vi "Launcher.vi"() -> ()   [LabVIEW 2020]
uses:
  <vilib>/Utility/miscctls.llb/LVPointTypeDef.ctl
  Controls/(Ctrl)Launcher_State Machine.ctl
  Controls/(Ctrl)Launcher_RedNoah3 Edition.ctl
  SubVIs/Control Data/Controls/(Ctrl)Control Data_Save or Load Control Data_Function.ctl
  SubVIs/Serial/Controls/(Ctrl)Serial_FGV Function.ctl
  <vilib>/Utility/sysdir.llb/System Directory Type.ctl
  SubVIs/Launcher/Controls/(Ctrl)Launcher_Edition Check form File_Function.ctl
  7ecfc601-dc53-4076-97e2-4cf976eadafe.vi
  31a6a614-1fdf-4bf0-963f-4008c2f34b95.vi
  <vilib>/security/Message Digest/API/Instances/File/SHA-256 File Checksum.vi
  <vilib>/httpClient/LabVIEWHTTPClient.lvlib
  <vilib>/zip/NI_Unzip.lvlib
  <vilib>/security/Message Digest/API/NI_Message Digest API.lvlib
panel:
  out "F/w Version":string
  out "Version":string
  out "Status":string
  # "Haptic Studio"
  # "with RedNoah3"
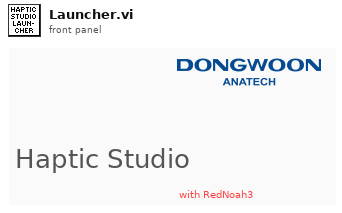
[diagram p1: front panel]
types:
  T1 = typedef "(Ctrl)Launcher_RedNoah3 Edition.ctl" = enum16{"Unknown", "Single Board", "Sensor Package"}
  T2 = typedef "(Ctrl)Launcher_State Machine.ctl" = enum16{"Check GUI Ver", "Update GUI", "Connect to BD", "Check FW Ver", "Update FW", "Check Edition", "Launch", "Server Connection Error", "BD Connection Error", "FW Update Error"}
  T3 = typedef "LVPointTypeDef.ctl" = cluster{"Horizontal":i16, "Vertical":i16}
  T4 = typedef "(Ctrl)Control Data_Save or Load Control Data_Function.ctl" = enum16{"Save", "Load"}
  T5 = cluster{"Major":i32, "Minor":i32, "Patch":i32, "Build":i32}
  T6 = typedef "(Ctrl)Serial_FGV Function.ctl" = enum16{"Initialize", "Read", "Read All", "Write", "Flush Buffer", "Get Ref.", "Close"}
  T7 = typedef "(Ctrl)Launcher_Edition Check form File_Function.ctl" = enum16{"Read", "Write"}
  T8 = enum32{"Invalid", "Standard", "Closed", "Hidden", "Minimized", "Maximized"}
  T9 = typedef "LabVIEWHTTPClient.lvlib/ClientHandle.ctl" = refnum<k1>
  T10 = typedef "Haptic IC.lvclass/(Ctrl)IC Type.ctl" = enum8{"DW7800", "DW7802", "DW7912", "DW7914"}
  T11 = cluster{"BD SN":string, "BD FW Version":u32, "BD HW Version":enum8{"BBB 1.0", "BBB 1.1", "WBB 1.0", "reserved", "RedNoah3"}}
  T12 = typedef "System Directory Type.ctl" = i32
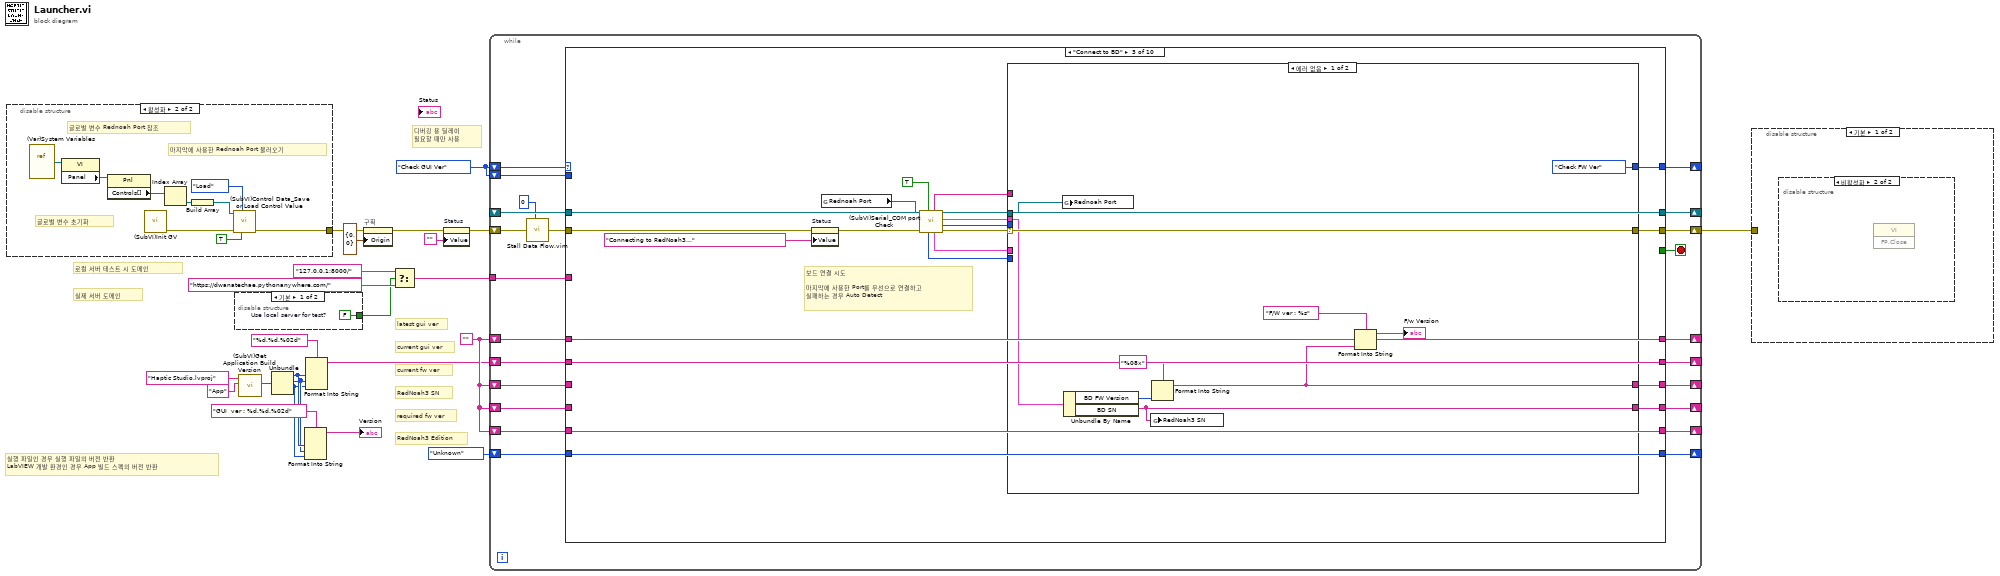
[diagram p0: block diagram]
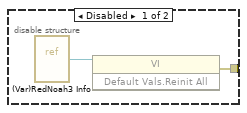
[diagram p2: hidden frame]
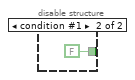
[diagram p3: hidden frame]
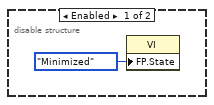
[diagram p4: hidden frame]
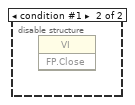
[diagram p5: hidden frame]
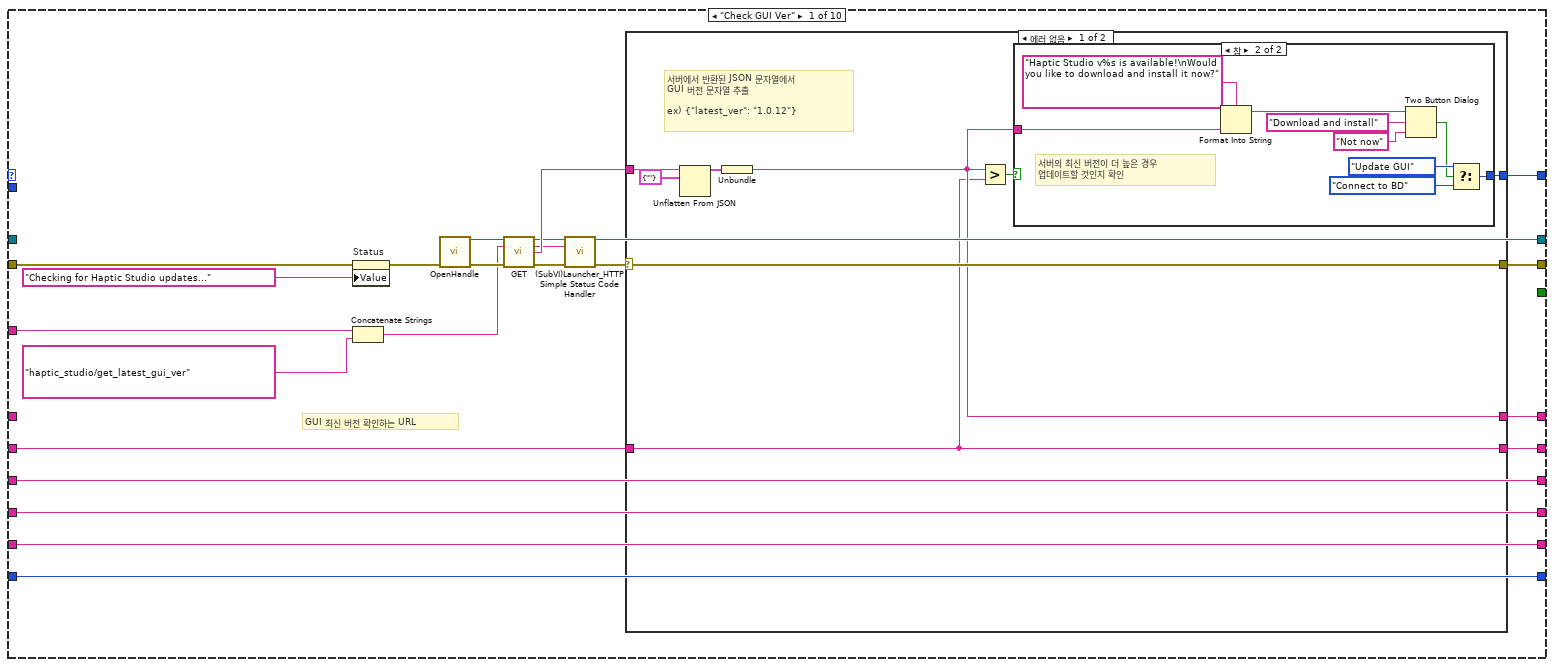
[diagram p6: hidden frame]
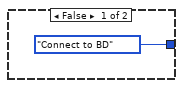
[diagram p7: hidden frame]
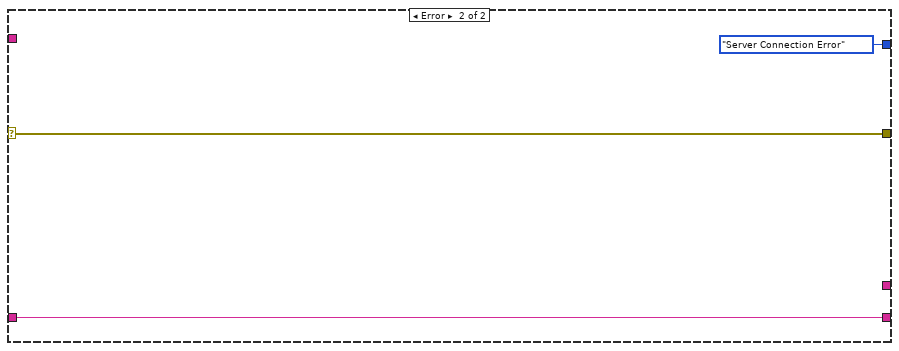
[diagram p8: hidden frame]
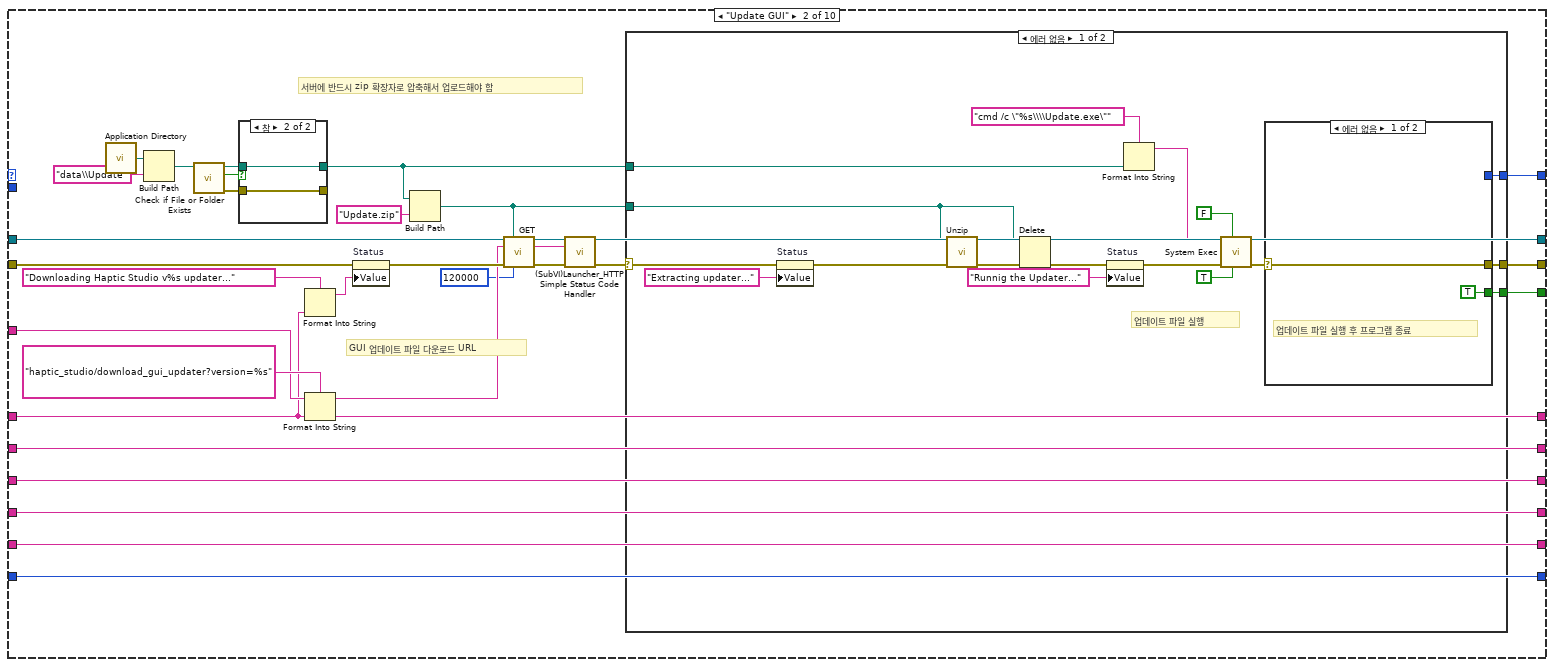
[diagram p9: hidden frame]
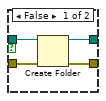
[diagram p10: hidden frame]
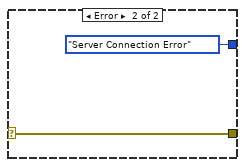
[diagram p11: hidden frame]
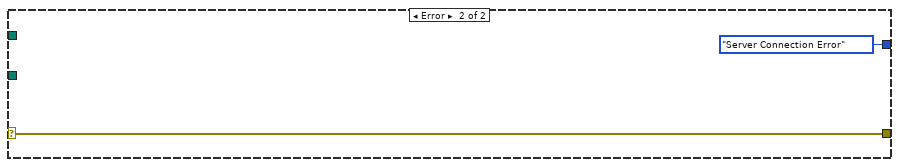
[diagram p12: hidden frame]
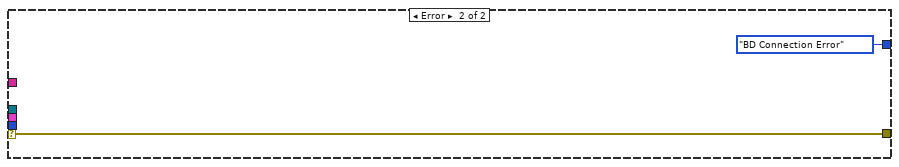
[diagram p13: hidden frame]
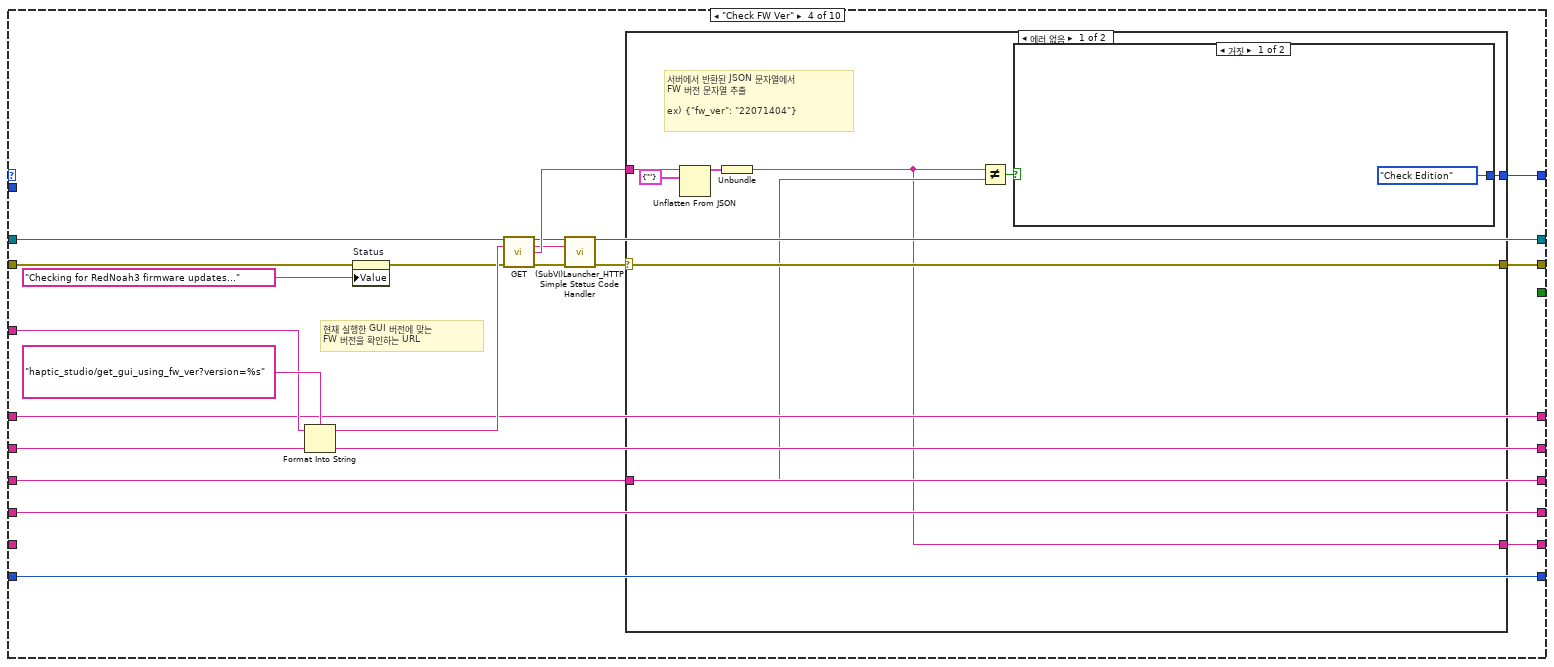
[diagram p14: hidden frame]
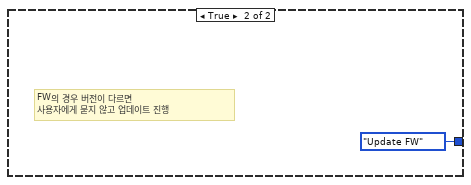
[diagram p15: hidden frame]
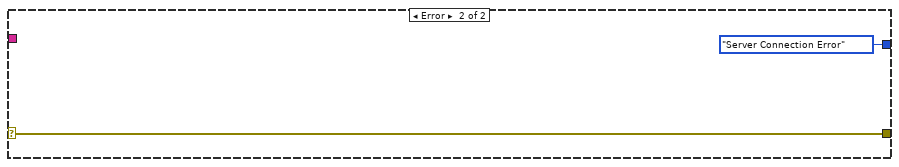
[diagram p16: hidden frame]
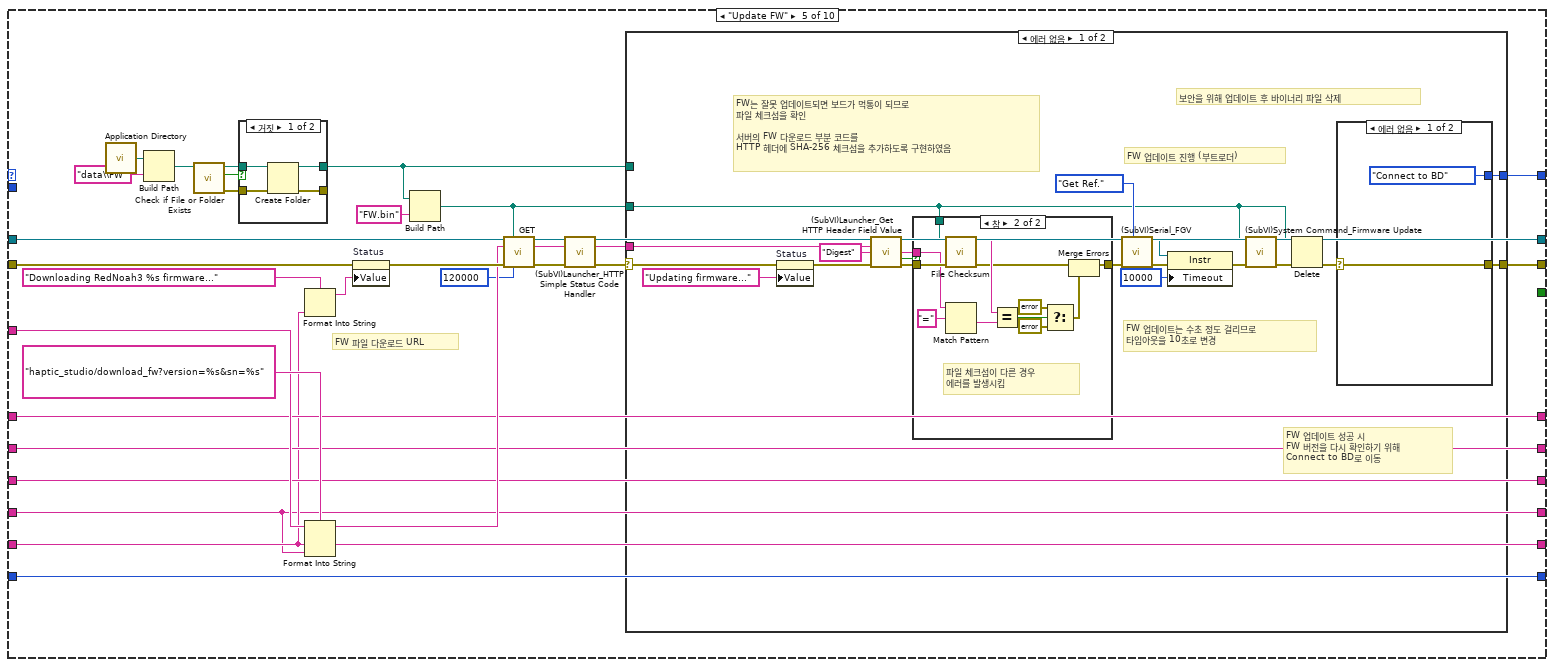
[diagram p17: hidden frame]
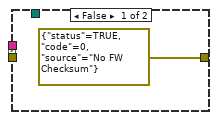
[diagram p19: hidden frame]
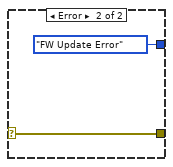
[diagram p20: hidden frame]
diagram:
  w16 = ""
  w15 = (Ctrl)Launcher_State_Machine."Check GUI Ver"
  # "실행 파일인 경우 실행 파일의 버전 반환\nLabVIEW 개발 환경인 경우 App 빌드 스펙의 버전 반환"
  # "디버깅 용 딜레이\n필요할 때만 사용"
  # "로컬 서버 테스트 시 도메인"
  # "실제 서버 도메인"
  # "RedNoah3 Edition"
  # "RedNoah3 SN"
  # "required fw ver"
  # "current fw ver"
  # "current gui ver"
  # "latest gui ver"
  n1 = disable-structure shown="활성화" {
    disable-tunnel: [w24 w33] -> w14
    frame Disabled {
      n2 = vi-ref "(Var)RedNoah3 Info.vi"() -> (w25:refnum<vi>)
      n3 = invoke class="VI" method="Default Vals.Reinit All"(reference=w25) -> (error out=w24:errorcluster)  [unwired: 2 in, 2 out]
    }
    frame Enabled {
      # "글로벌 변수 Rednoah Port 참조"
      # "마지막에 사용한 Rednoah Port 불러오기"
      # "글로벌 변수 초기화"
      n4 = vi-ref "(Var)System Variables.vi"() -> (w32:refnum<vi>)
      n5 = property class="VI"(reference=w32) -> ("Panel"=w31:refnum<vi>)  [unwired: 1 in, 2 out]
      n6 = property class="Pnl"(reference=w31) -> ("Controls[]"=w30:refnum<vi>[])  [unwired: 1 in, 2 out]
      n7 = call "(SubVI)Init GV.vi"() -> ("error out"=w34:errorcluster)  [unwired: 11 in]
      n8 = Index Array(array=w30) -> (element=w29:refnum<vi>)  [unwired: 1 in]
      n9 = Build Array(w29) -> (w28:refnum<vi>[])
      n10 = call "(SubVI)Control Data_Save or Load Control Value.vi"("Common? (f)"=TRUE, "Function"=(Ctrl)Control_Data_Save_or_Load_Control_Data_Function."Load", "error in (no error)"=w34, "Control Ref"=w28) -> ("error out"=w33:errorcluster)  [unwired: 7 in]
    }
  }
  n11 = disable-structure shown="기본" {
    disable-tunnel: [w35 FALSE ("s")] -> w19
    frame condition #0 (active) {
      w35 = FALSE  # Use local server for test?
    }
    frame condition #1 {
    }
  }
  n12 = call "(SubVI)Get Application Build Version.vi"("Build Specification Name"="App", "Project Filename"="Haptic Studio.lvproj") -> ("Version Numbers"=w10:T5)  [unwired: 7 in, 2 out]
  n13 = Unbundle(w10) -> ("Major"=w4:i32, "Minor"=w2:i32, "Patch"=w1:i32)  [unwired: 1 out]
  n14 = Format Into String(format string="GUI  ver : %d.%d.%02d" ("포맷 문자열"), w4, w2, w1) -> (resulting string=→"Version":string)  [unwired: 2 in, 1 out]
  n15 = Format Into String(format string="%d.%d.%02d" ("포맷 문자열"), w4, w2, w1) -> (resulting string=w6:string)  [unwired: 2 in, 1 out]
  n16 = property on="구획" class="Pane"(error in=w14, "Origin"=T3 {"Horizontal"=0, "Vertical"=0} ("원점")) -> (error out=w13:errorcluster)  [unwired: 1 in, 1 out]
  n17 = Select(t="127.0.0.1:8000/", s=w19, f="https://dwanatechae.pythonanywhere.com/") -> (s? t:f=w18:string)
  n18 = property on="Status" class="Str"(error in=w13, "Value"="" ("Status")) -> (error out=w11:errorcluster)  [unwired: 1 in, 1 out]
  n19 = while {
    shift-right: [w40] -> w22
    shift-left: w11 -> [w59]
    shift-right: [w57] -> _
    shift-left: _ -> [w56]
    shift-right: [w55] -> _
    shift-left: w16 -> [w54]
    shift-right: [w53] -> _
    shift-left: w15 -> [w58]
    tunnel: w18 -> [w51]
    shift-right: [w50] -> _
    shift-left: w6 -> [w49]
    shift-right: [w48] -> _
    shift-left: w16 -> [w37]
    shift-right: [w47] -> _
    shift-left: w16 -> [w46]
    shift-right: [w45] -> _
    shift-left: w16 -> [w44]
    shift-right: [w43] -> _
    shift-left: (Ctrl)Launcher_RedNoah3_Edition."Unknown" -> [w42]
    shift-left: w15 -> [w41]
    stop <- w52 stop-if-true
    n20 = call "Stall Data Flow.vim"("value in"=w59, "milliseconds to wait"=u32 0) -> ("value out"=w39:errorcluster)  [unwired: 1 out]
    n21 = case shown="\"Connect to BD\"" w58 {
      selector: w58 -> [_ _ _ _ _ _ _ w383 w401 w420]
      tunnel: w39 -> [w80 w135 w185 w218 w262 w329 w346 w387 w415 w434]
      tunnel: [w75 w132 w182 w214 w259 w324 w353 _ _ _] -> w40
      tunnel: [w62 w105 w180 w199 w234 w309 w359 w391 w419 w438] -> w57
      tunnel: w56 -> [_ w130 w180 w204 w257 _ w359 w391 w419 w438]
      tunnel: [w74 w108 w168 w207 w241 w319 w358 w390 w418 w437] -> w55
      tunnel: w54 -> [_ w108 w168 w207 w241 w319 w358 w390 w418 w437]
      tunnel: [w77 w134 w184 w216 w261 w326 _ w380 w405 w424] -> w53
      tunnel: [_ w115 _ _ _ _ TRUE _ _ _] -> w52
      tunnel: w51 -> [w73 w114 _ w212 w242 w322 _ _ _ _]
      tunnel: [w70 w113 w169 w208 w240 w317 w357 w389 w417 w436] -> w50
      tunnel: w49 -> [w60 w113 w169 w208 w240 w317 w357 w389 w417 w436]
      tunnel: [w69 w112 w171 w205 w239 w316 w352 w385 w413 w432] -> w48
      tunnel: w37 -> [w69 w112 _ w205 w239 w316 w352 w385 w413 w432]
      tunnel: [w67 w110 w167 w210 w237 w318 w356 w388 w416 w435] -> w47
      tunnel: w46 -> [w67 w110 w167 _ w237 w318 w356 w388 w416 w435]
      tunnel: [w68 w111 w170 w209 w231 w307 w351 w381 w412 w431] -> w45
      tunnel: w44 -> [w68 w111 _ w209 w231 w307 w351 w381 w412 w431]
      tunnel: [w66 w109 w166 w206 w238 w320 w350 w378 w411 w430] -> w43
      tunnel: w42 -> [w66 w109 w166 w206 w238 _ w350 w379 w411 w430]
      tunnel: w41 -> [_ _ _ _ _ _ _ w382 w402 w421]
      frame "Check GUI Ver" {
        # "GUI 최신 버전 확인하는 URL"
        n22 = property on="Status" class="Str"(error in=w80, "Value"="Checking for Haptic Studio updates..." ("Status")) -> (error out=w79:errorcluster)  [unwired: 1 in, 1 out]
        n23 = Concatenate Strings(w73, "haptic_studio/get_latest_gui_ver" ("url")) -> (w71:string)
        n24 = call <vilib>:"OpenHandle.vi"("error in (no error)"=w79) -> ("client handle out"=w82:T9, "error out"=w81:errorcluster)  [unwired: 13 in]
        n25 = call <vilib>:"GET.vi"("client handle"=w82, "url"=w71, "error in (no error)"=w81) -> ("client handle out"=w63:T9, "headers"=w61:string, "body"=w65:string, "error out"=w76:errorcluster)  [unwired: 9 in]
        n26 = call "(SubVI)Launcher_HTTP Simple Status Code Handler.vi"("client handle in"=w63, "HTTP Header"=w61, "error in (no error)"=w76) -> ("client handle out"=w62:T9, "error out"=w64:errorcluster)  [unwired: 7 in, 4 out]
        n27 = case shown="에러 없음" w64 {
          selector: w64 -> [w85 w103]
          tunnel: w65 -> [w88 _]
          tunnel: [w86 (Ctrl)Launcher_State_Machine."Server Connection Error" ("f")] -> w77
          tunnel: [w85 w103] -> w75
          tunnel: [w84 _] -> w74
          tunnel: [w83 w101] -> w70
          tunnel: w60 -> [w83 w101]
          frame No Error {
            # "서버에서 반환된 JSON 문자열에서\nGUI 버전 문자열 추출\n\nex) {\"latest_ver\": \"1.0.12\"}"
            n28 = Unflatten From JSON(JSON string=w88, type and defaults=cluster{"latest_ver":string} {"latest_ver"=""}) -> (value=w89:cluster{"latest_ver":string})  [unwired: 5 in, 1 out]
            n29 = Unbundle(w89) -> ("latest_ver"=w84:string)
            n30 = Greater?(x=w84, y=w83) -> (0:w87:bool)
            n31 = case shown="참" w87 {
              tunnel: [(Ctrl)Launcher_State_Machine."Connect to BD" ("f") w98] -> w86
              tunnel: w84 -> [_ w92]
              frame False {
              }
              frame True {
                # "서버의 최신 버전이 더 높은 경우\n업데이트할 것인지 확인"
                n32 = Format Into String(format string="Haptic Studio v%s is available!\nWould you like to download and install it now?" ("메시지"), w92) -> (resulting string=w95:string)  [unwired: 2 in, 1 out]
                n33 = Two Button Dialog(message=w95, 1:"Not now" ("거짓 버튼 이름(\"취소\")"), 2:"Download and install" ("참 버튼 이름(\"확인\")")) -> (T button?=w97:bool)
                n34 = Select(t=(Ctrl)Launcher_State_Machine."Update GUI", s=w97, f=(Ctrl)Launcher_State_Machine."Connect to BD") -> (s? t:f=w98:T2)
              }
            }
          }
          frame Error {
          }
        }
      }
      frame "Update GUI" {
        # "서버에 반드시 zip 확장자로 압축해서 업로드해야 함"
        # "GUI 업데이트 파일 다운로드 URL"
        n35 = call <vilib>:"Application Directory.vi"() -> ("Application Directory"=w125:path)
        n36 = Build Path(base path=w125, name or relative path="data\\Update" ("이름 또는 상대 경로")) -> (appended path=w123:path)
        n37 = call <vilib>:"Check if File or Folder Exists.vi"("path"=w123) -> ("error out"=w121:errorcluster, "file or folder exists?"=w122:bool, "dup path"=w120:path)  [unwired: 8 in]
        n38 = case shown="참" w122 {
          tunnel: w121 -> [w139 w141]
          tunnel: [w138 w141] -> _
          tunnel: w120 -> [w137 w140]
          tunnel: [w136 w140] -> w116
          frame False {
            n39 = Create Folder(path (use dialog)=w137, error in=w139) -> (created path=w136:path, error out=w138:errorcluster)  [unwired: 1 in, 1 out]
          }
          frame True {
          }
        }
        n40 = Format Into String(format string="Downloading Haptic Studio v%s updater..." ("Status"), w108) -> (resulting string=w128:string)  [unwired: 2 in, 1 out]
        n41 = Format Into String(format string="haptic_studio/download_gui_updater?version=%s" ("url"), initial string=w114, w108) -> (resulting string=w126:string)  [unwired: 1 in, 1 out]
        n42 = property on="Status" class="Str"(error in=w135, "Value"=w128) -> (error out=w131:errorcluster)  [unwired: 1 in, 1 out]
        n43 = Build Path(base path=w116, name or relative path="Update.zip" ("이름 또는 상대 경로")) -> (appended path=w117:path)
        n44 = call <vilib>:"GET.vi"("client handle"=w130, "output file"=w117, "url"=w126, "error in (no error)"=w131, "timeout (10000)"=120000) -> ("client handle out"=w106:T9, "headers"=w104:string, "error out"=w133:errorcluster)  [unwired: 7 in, 1 out]
        n45 = call "(SubVI)Launcher_HTTP Simple Status Code Handler.vi"("client handle in"=w106, "HTTP Header"=w104, "error in (no error)"=w133) -> ("client handle out"=w105:T9, "error out"=w107:errorcluster)  [unwired: 7 in, 4 out]
        n46 = case shown="에러 없음" w107 {
          selector: w107 -> [w150 w164]
          tunnel: [w142 (Ctrl)Launcher_State_Machine."Server Connection Error" ("f")] -> w134
          tunnel: [w143 w164] -> w132
          tunnel: w117 -> [w157 _]
          tunnel: w116 -> [w156 _]
          tunnel: [w152 _] -> w115
          frame No Error {
            # "업데이트 파일 실행"
            n47 = property on="Status" class="Str"(error in=w150, "Value"="Extracting updater..." ("Status")) -> (error out=w149:errorcluster)  [unwired: 1 in, 1 out]
            n48 = call <vilib>:"Unzip.vi"("error in (no error)"=w149, "Zip file"=w157) -> ("error out"=w158:errorcluster)  [unwired: 7 in, 2 out]
            n49 = Delete(path (use dialog)=w157, error in=w158) -> (error out=w146:errorcluster)  [unwired: 3 in, 2 out]
            n50 = property on="Status" class="Str"(error in=w146, "Value"="Runnig the Updater..." ("Status")) -> (error out=w145:errorcluster)  [unwired: 1 in, 1 out]
            n51 = Format Into String(format string="cmd /c \"%s\\\\Update.exe\"" ("포맷 문자열"), w156) -> (resulting string=w154:string)  [unwired: 2 in, 1 out]
            n52 = call <vilib>:"System Exec.vi"("run minimized? (F)"=TRUE, "wait until completion? (T)"=FALSE, "error in (no error)"=w145, "command line"=w154) -> ("error out"=w144:errorcluster)  [unwired: 4 in, 3 out]
            n53 = case shown="에러 없음" w144 {
              selector: w144 -> [w160 w162]
              tunnel: [TRUE _] -> w152
              tunnel: [w160 w162] -> w143
              tunnel: [_ (Ctrl)Launcher_State_Machine."Server Connection Error" ("f")] -> w142
              frame No Error {
                # "업데이트 파일 실행 후 프로그램 종료"
              }
              frame Error {
              }
            }
          }
          frame Error {
          }
        }
      }
      frame "Connect to BD" {
        # "보드 연결 시도\n\n마지막에 사용한 Port를 우선으로 연결하고\n실패하는 경우 Auto Detect"
        n54 = property on="Status" class="Str"(error in=w185, "Value"="Connecting to RedNoah3..." ("Status")) -> (error out=w181:errorcluster)  [unwired: 1 in, 1 out]
        n55 = global read "(Var)System Variables.vi" "Rednoah Port"() -> (w165:refnum<visa-resource-name>)
        n56 = call "(SubVI)Serial_COM port Check.vi"("Auto Detect?"=TRUE, "error in (no error)"=w181, "VISA resource name"=w165) -> ("error out"=w183:errorcluster, "IC Type"=w173:T10, "BD Version"=w175:T11, "VISA resource name out"=w174:refnum<visa-resource-name>, "I2C Slave ID"=w177:cluster{string, u8}[], "BD Info Str"=w178:string, "Default I2C Slave ID"=w176:u8)  [unwired: 2 in]
        n57 = case shown="에러 없음" w183 {
          selector: w183 -> [w194 w197]
          tunnel: [(Ctrl)Launcher_State_Machine."Check FW Ver" ("f") (Ctrl)Launcher_State_Machine."BD Connection Error" ("f")] -> w184
          tunnel: [w194 w197] -> w182
          tunnel: w178 -> [_ _]
          tunnel: w177 -> [_ _]
          tunnel: w176 -> [_ _]
          tunnel: w175 -> [w193 _]
          tunnel: w174 -> [w189 _]
          tunnel: w173 -> [_ _]
          tunnel: [w187 _] -> w171
          tunnel: [w190 _] -> w170
          frame No Error {
            n58 = global write "(Var)System Variables.vi" "Rednoah Port"(w189) -> ()
            n59 = Unbundle By Name(w193) -> ("BD FW Version"=w192:u32, "BD SN"=w190:string)
            n60 = global write "(Var)RedNoah3 Info.vi" "RedNoah3 SN"(w190) -> ()
            n61 = Format Into String(format string="%08x" ("포맷 문자열"), w192) -> (resulting string=w187:string)  [unwired: 2 in, 1 out]
            n62 = Format Into String(format string="F/W ver : %s" ("포맷 문자열"), w187) -> (resulting string=→"F/w Version":string)  [unwired: 2 in, 1 out]
          }
          frame Error {
          }
        }
      }
      frame "Check FW Ver" {
        # "현재 실행한 GUI 버전에 맞는 \nFW 버전을 확인하는 URL"
        n63 = Format Into String(format string="haptic_studio/get_gui_using_fw_ver?version=%s" ("url"), initial string=w212, w208) -> (resulting string=w211:string)  [unwired: 1 in, 1 out]
        n64 = property on="Status" class="Str"(error in=w218, "Value"="Checking for RedNoah3 firmware updates..." ("Status")) -> (error out=w203:errorcluster)  [unwired: 1 in, 1 out]
        n65 = call <vilib>:"GET.vi"("client handle"=w204, "url"=w211, "error in (no error)"=w203) -> ("client handle out"=w200:T9, "headers"=w198:string, "body"=w202:string, "error out"=w215:errorcluster)  [unwired: 9 in]
        n66 = call "(SubVI)Launcher_HTTP Simple Status Code Handler.vi"("client handle in"=w200, "HTTP Header"=w198, "error in (no error)"=w215) -> ("client handle out"=w199:T9, "error out"=w201:errorcluster)  [unwired: 7 in, 4 out]
        n67 = case shown="에러 없음" w201 {
          selector: w201 -> [w221 w230]
          tunnel: w202 -> [w224 _]
          tunnel: [w222 (Ctrl)Launcher_State_Machine."Server Connection Error" ("f")] -> w216
          tunnel: [w221 w230] -> w214
          tunnel: w205 -> [w220 _]
          tunnel: [w219 _] -> w210
          frame No Error {
            # "서버에서 반환된 JSON 문자열에서\nFW 버전 문자열 추출\n\nex) {\"fw_ver\": \"22071404\"}"
            n68 = Unflatten From JSON(JSON string=w224, type and defaults=cluster{"fw_ver":string} {"fw_ver"=""}) -> (value=w225:cluster{"fw_ver":string})  [unwired: 5 in, 1 out]
            n69 = Unbundle(w225) -> ("fw_ver"=w219:string)
            n70 = Not Equal?(x=w219, y=w220) -> (x != y?=w223:bool)
            n71 = case shown="거짓" w223 {
              tunnel: [(Ctrl)Launcher_State_Machine."Check Edition" ("f") (Ctrl)Launcher_State_Machine."Update FW" ("f")] -> w222
              frame False {
              }
              frame True {
                # "FW의 경우 버전이 다르면\n사용자에게 묻지 않고 업데이트 진행"
              }
            }
          }
          frame Error {
          }
        }
      }
      frame "Update FW" {
        # "FW 파일 다운로드 URL"
        n72 = call <vilib>:"Application Directory.vi"() -> ("Application Directory"=w252:path)
        n73 = Build Path(base path=w252, name or relative path="data\\FW" ("이름 또는 상대 경로")) -> (appended path=w250:path)
        n74 = call <vilib>:"Check if File or Folder Exists.vi"("path"=w250) -> ("error out"=w248:errorcluster, "file or folder exists?"=w249:bool, "dup path"=w247:path)  [unwired: 8 in]
        n75 = case shown="거짓" w249 {
          tunnel: w248 -> [w266 w268]
          tunnel: [w265 w268] -> _
          tunnel: w247 -> [w264 w267]
          tunnel: [w263 w267] -> w243
          frame False {
            n76 = Create Folder(path (use dialog)=w264, error in=w266) -> (created path=w263:path, error out=w265:errorcluster)  [unwired: 1 in, 1 out]
          }
          frame True {
          }
        }
        n77 = Format Into String(format string="Downloading RedNoah3 %s firmware..." ("Status"), w237) -> (resulting string=w255:string)  [unwired: 2 in, 1 out]
        n78 = Format Into String(format string="haptic_studio/download_fw?version=%s&sn=%s" ("url"), initial string=w242, w237, w231) -> (resulting string=w253:string)  [unwired: 1 in, 1 out]
        n79 = property on="Status" class="Str"(error in=w262, "Value"=w255) -> (error out=w258:errorcluster)  [unwired: 1 in, 1 out]
        n80 = Build Path(base path=w243, name or relative path="FW.bin" ("이름 또는 상대 경로")) -> (appended path=w244:path)
        n81 = call <vilib>:"GET.vi"("client handle"=w257, "output file"=w244, "url"=w253, "error in (no error)"=w258, "timeout (10000)"=120000) -> ("client handle out"=w235:T9, "headers"=w233:string, "error out"=w260:errorcluster)  [unwired: 7 in, 1 out]
        n82 = call "(SubVI)Launcher_HTTP Simple Status Code Handler.vi"("client handle in"=w235, "HTTP Header"=w233, "error in (no error)"=w260) -> ("client handle out"=w234:T9, "Header"=w232:string, "error out"=w236:errorcluster)  [unwired: 7 in, 3 out]
        n83 = case shown="에러 없음" w236 {
          selector: w236 -> [w277 w306]
          tunnel: [w285 (Ctrl)Launcher_State_Machine."Server Connection Error" ("f")] -> w261
          tunnel: [w286 w306] -> w259
          tunnel: w244 -> [w270 _]
          tunnel: w243 -> [_ _]
          tunnel: w232 -> [w275 _]
          frame No Error {
            # "FW 업데이트 성공 시 \nFW 버전을 다시 확인하기 위해\nConnect to BD로 이동"
            # "보안을 위해 업데이트 후 바이너리 파일 삭제"
            # "FW 업데이트 진행 (부트로더)"
            # "FW 업데이트는 수초 정도 걸리므로\n타임아웃을 10초로 변경"
            # "FW는 잘못 업데이트되면 보드가 먹통이 되므로\n파일 체크섬을 확인\n\n서버의 FW 다운로드 부분 코드를\nHTTP 헤더에 SHA-256 체크섬을 추가하도록 구현하였음"
            n84 = property on="Status" class="Str"(error in=w277, "Value"="Updating firmware..." ("Status")) -> (error out=w276:errorcluster)  [unwired: 1 in, 1 out]
            n85 = call "(SubVI)Launcher_Get HTTP Header Field Value.vi"("Header in"=w275, "Field"="Digest", "error in (no error)"=w276) -> ("Value"=w271:string, "Found?"=w272:bool, "error out"=w274:errorcluster)  [unwired: 8 in, 2 out]
            n86 = case shown="참" w272 {
              tunnel: w274 -> [_ w300]
              tunnel: [errorcluster {"status"=TRUE, "code"=0, "source"="No FW Checksum"} ("error IO") w292] -> w273
              tunnel: w271 -> [_ w298]
              tunnel: w270 -> [_ w299]
              frame False {
              }
              frame True {
                # "파일 체크섬이 다른 경우\n에러를 발생시킴"
                n87 = call-poly <vilib>:"File Checksum.vi"("error in"=w300, "path"=w299) -> ("error out"=w293:errorcluster, "digest"=w295:string)  [unwired: 8 in]
                n88 = Match Pattern(string=w298, regular expression="=" ("정규식")) -> (after substring=w296:string)  [unwired: 1 in, 3 out]
                n89 = Equal?(x=w295, y=w296) -> (x = y?=w294:bool)
                n90 = Select(t=errorcluster {"status"=FALSE, "code"=0, "source"=""}, s=w294, f=errorcluster {"status"=TRUE, "code"=0, "source"="FW Checksum Error"} ("에러 상수")) -> (s? t:f=w289:errorcluster)
                n91 = Merge Errors(w293, w289) -> (w292:errorcluster)
              }
            }
            n92 = call "(SubVI)Serial_FGV.vi"("Function"=(Ctrl)Serial_FGV_Function."Get Ref.", "error in (no error)"=w273) -> ("error out"=w283:errorcluster, "VISA resource name out"=w280:refnum<visa-resource-name>)  [unwired: 7 in, 1 out]
            n93 = property class="Instr"(reference=w280, error in=w283, "Timeout"=u32 10000 ("General Settings:Timeout Value")) -> (error out=w281:errorcluster)  [unwired: 1 out]
            n94 = call "(SubVI)System Command_Firmware Update.vi"("error in (no error)"=w281, "FW File"=w270) -> ("error out"=w269:errorcluster)  [unwired: 8 in, 1 out]
            n95 = Delete(path (use dialog)=w270, error in=w269) -> (error out=w284:errorcluster)  [unwired: 3 in, 2 out]
            n96 = case shown="에러 없음" w284 {
              selector: w284 -> [w302 w304]
              tunnel: [w302 w304] -> w286
              tunnel: [(Ctrl)Launcher_State_Machine."Connect to BD" ("f") (Ctrl)Launcher_State_Machine."FW Update Error" ("f")] -> w285
              frame No Error {
              }
              frame Error {
              }
            }
          }
          frame Error {
          }
        }
      }
      frame "Check Edition" {
        w315 = T12 0 items=["사용자 홈"=0, "사용자 데스크탑"=1, "사용자 문서"=2, "사용자 어플리케이션 데이터"=3, "사용자 환경"=4, "사용자 임시"=5, "퍼블릭 문서"=6, "퍼블릭 어플리케이션 데이터"=7, "퍼블릭 환경"=8, "퍼블릭 캐시"=13, "시스템 코어 라이브러리"=9, "시스템 설치된 라이브러리"=10, "어플리케이션 파일"=11, "부팅 볼륨 루트"=12] ("system directory type")
        # "RedNoah3 S/N로 에디션을 확인하는 URL"
        n97 = call <vilib>:"Get System Directory.vi"("system directory type"=w315) -> ("system directory"=w314:path)  [unwired: 10 in]
        n98 = Strip Path(path=w314) -> (name=w313:string)  [unwired: 1 out]
        n99 = Format Into String(format string="haptic_studio/get_rednoah_edition?sn=%s&fw_version=%s&user=%s" ("url"), initial string=w322, w307, w316, w313) -> (resulting string=w321:string)  [unwired: 1 in, 1 out]
        n100 = property on="Status" class="Str"(error in=w329, "Value"="Checking the RedNoah3 edition..." ("Status")) -> (error out=w328:errorcluster)  [unwired: 1 in, 1 out]
        n101 = call <vilib>:"OpenHandle.vi"("error in (no error)"=w328) -> ("client handle out"=w331:T9, "error out"=w330:errorcluster)  [unwired: 13 in]
        n102 = call <vilib>:"GET.vi"("client handle"=w331, "url"=w321, "error in (no error)"=w330) -> ("client handle out"=w310:T9, "headers"=w308:string, "body"=w312:string, "error out"=w325:errorcluster)  [unwired: 9 in]
        n103 = call "(SubVI)Launcher_HTTP Simple Status Code Handler.vi"("client handle in"=w310, "HTTP Header"=w308, "error in (no error)"=w325) -> ("client handle out"=w309:T9, "error out"=w311:errorcluster)  [unwired: 7 in, 4 out]
        n104 = case shown="에러 없음" w311 {
          selector: w311 -> [w339 w344]
          tunnel: w312 -> [w340 _]
          tunnel: [(Ctrl)Launcher_State_Machine."Launch" ("f") (Ctrl)Launcher_State_Machine."Server Connection Error" ("f")] -> w326
          tunnel: [w339 w344] -> w324
          tunnel: [w333 _] -> w320
          tunnel: w307 -> [w334 _]
          frame No Error {
            # "인터넷 연결되지 않았을 때를 대비해\nSensor Package인 경우 S/N를 저장"
            n105 = Unflatten From JSON(JSON string=w340, type and defaults=cluster{"edition":string} {"edition"=""}) -> (value=w341:cluster{"edition":string})  [unwired: 5 in, 1 out]
            n106 = Unbundle(w341) -> ("edition"=w338:string)
            n107 = Scan From String(input string=w338, default 1=(Ctrl)Launcher_RedNoah3_Edition."Unknown") -> (error out=w336:errorcluster, output 1=w333:T1)  [unwired: 3 in, 2 out]
            n108 = global write "(Var)RedNoah3 Info.vi" "RedNoah3 Edition"(w333) -> ()
            n109 = call <vilib>:"Clear Errors.vi"("error in (no error)"=w336) -> ()  [unwired: 5 in, 2 out]
            n110 = call "(SubVI)Launcher_Edition Check from File.vi"("Function"=(Ctrl)Launcher_Edition_Check_form_File_Function."Write", "SN"=w334, "Edition in"=w333) -> ()  [unwired: 8 in, 1 out]
          }
          frame Error {
          }
        }
      }
      frame "Launch", Default {
        # "자연스럽게 실행으로 넘어가기 위한 딜레이\n지워도 무방함"
        n111 = case shown="에러 없음" w346 {
          selector: w346 -> [w360 _]
          tunnel: [w360 _] -> w345
          frame No Error {
            n112 = global write "(Var)System Variables.vi" "Quit System"(TRUE ("Quit System")) -> ()
          }
          frame Error {
          }
        }
        n113 = property on="Status" class="Str"(error in=w345, "Value"="Loading Haptic Stuidio..." ("Status")) -> (error out=w354:errorcluster)  [unwired: 1 in, 1 out]
        n114 = call "Stall Data Flow.vim"("value in"=w354, "milliseconds to wait"=u32 500) -> ("value out"=w349:errorcluster)  [unwired: 1 out]
        n115 = disable-structure shown="활성화" {
          disable-tunnel: w349 -> [w368 w370]
          disable-tunnel: [w367 w376] -> w353
          frame Disabled {
            w366 = FALSE ("완료될 때까지 기다림")
            n116 = vi-ref "Main.vi"() -> (w369:refnum<vi>)
            n117 = invoke class="VI" method="Run VI"(reference=w369, error in=w368, "Wait until done"=w366, "Auto Dispose Ref"=w366) -> (reference out=w365:refnum<vi>, error out=w364:errorcluster)  [unwired: 1 in, 3 out]
            n118 = invoke class="VI" method="FP.Open"(reference=w365, error in=w364, "Activate"=TRUE ("활성화?"), "State"=T8."Standard" ("상태")) -> (error out=w367:errorcluster)  [unwired: 1 in, 4 out]
          }
          frame Enabled {
            n119 = vi-ref "Main.vi"() -> (w377:refnum<vi>)
            n120 = property class="VI 인터페이스 타입 0"(reference=w377, error in=w370) -> (reference out=w374:refnum<vi>, "Name"=w375:string)  [unwired: 1 out]
            n121 = Open VI Reference(type specifier VI Refnum (for type only)=w374, vi path=w375, options=128 ("옵션")) -> (vi reference=w372:refnum<vi>, error out=w371:errorcluster)  [unwired: 3 in]
            n122 = call-by-ref "비동기화 호출 시작"(reference=w372, error in=w371) -> (error out=w376:errorcluster)  [unwired: 12 in, 1 out]
          }
        }
      }
      frame "Server Connection Error" {
        # "에러 발생 시 디버깅이 용이하도록\n에러 내용을 저장"
        n123 = call "(SubVI)Launcher_Error Log.vi"("error in (no error)"=w387, "Previous State"=w382, "Error State"=w383) -> ("error out"=w384:errorcluster)  [unwired: 8 in]
        n124 = property on="Status" class="Str"(error in=w384, "Value"="Update server error..." ("Status")) -> ()  [unwired: 1 in, 2 out]
        n125 = case shown="\"Check Edition\"" w382 {
          tunnel: w381 -> [_ _ w399]
          tunnel: [(Ctrl)Launcher_State_Machine."Connect to BD" ("f") (Ctrl)Launcher_State_Machine."Check Edition" ("f") (Ctrl)Launcher_State_Machine."Launch" ("f")] -> w380
          tunnel: w379 -> [w392 w394 w398]
          tunnel: [w392 w394 w396] -> w378
          frame "Check GUI Ver", "Update GUI", Default {
          }
          frame "Check FW Ver", "Update FW" {
          }
          frame "Check Edition" {
            # "Check Edition 시도 중 서버 관련 에러 발생 시\n파일에서 S/N를 조회\nSensor Package만 저장되어 있음"
            n126 = call "(SubVI)Launcher_Edition Check from File.vi"("Function"=(Ctrl)Launcher_Edition_Check_form_File_Function."Read", "SN"=w399, "Edition in"=w398) -> ("Edition out"=w396:T1)  [unwired: 8 in]
            n127 = global write "(Var)RedNoah3 Info.vi" "RedNoah3 Edition"(w396) -> ()
          }
        }
      }
      frame "BD Connection Error" {
        # "에러 발생 시 디버깅이 용이하도록\n에러 내용을 저장"
        n128 = call "(SubVI)Launcher_Error Log.vi"("error in (no error)"=w415, "Previous State"=w402, "Error State"=w401) -> ("error out"=w403:errorcluster)  [unwired: 8 in]
        n129 = property on="Status" class="Str"(error in=w403, "Value"="RedNoah3 connection error..." ("Status")) -> ()  [unwired: 1 in, 2 out]
        n130 = Two Button Dialog(message="RedNoah3 not found.\nSome fuctions are limited.\n\nIf RedNoah3 is connected, \nplease reset or reconnect the borad and retry." ("메시지"), 1:"OK" ("거짓 버튼 이름(\"취소\")"), 2:"Retry" ("참 버튼 이름(\"확인\")")) -> (T button?=w404:bool)
        n131 = Select(t=(Ctrl)Launcher_State_Machine."Connect to BD" ("f"), s=w404, f=(Ctrl)Launcher_State_Machine."Launch") -> (s? t:f=w405:T2)
      }
      frame "FW Update Error" {
        # "에러 발생 시 디버깅이 용이하도록\n에러 내용을 저장"
        n132 = call "(SubVI)Launcher_Error Log.vi"("error in (no error)"=w434, "Previous State"=w421, "Error State"=w420) -> ("error out"=w422:errorcluster)  [unwired: 8 in]
        n133 = property on="Status" class="Str"(error in=w422, "Value"="RedNoah3 firmware update error..." ("Status")) -> ()  [unwired: 1 in, 2 out]
        n134 = Two Button Dialog(message="RedNoah3 firmware update failed.\nThis RedNoah may be for other software.\nSome fuctions are limited.\n\nIf the update continues to fail,\nplease contact to Dongwoon Anatech." ("메시지"), 1:"OK" ("거짓 버튼 이름(\"취소\")"), 2:"Retry" ("참 버튼 이름(\"확인\")")) -> (T button?=w423:bool)
        n135 = Select(t=(Ctrl)Launcher_State_Machine."Connect to BD" ("f"), s=w423, f=(Ctrl)Launcher_State_Machine."Check Edition") -> (s? t:f=w424:T2)
      }
    }
  }
  n136 = disable-structure shown="기본" {
    disable-tunnel: w22 -> [_ _]
    frame condition #0 (active) {
      n137 = disable-structure shown="비활성화" {
        frame Enabled {
          n138 = property class="VI"("FP.State"=T8."Minimized" ("프런트패널 윈도우:상태")) -> ()  [unwired: 2 in, 2 out]
        }
        frame Disabled {
          n139 = invoke class="VI" method="FP.Close"() -> ()  [unwired: 3 in, 3 out]
        }
      }
    }
    frame condition #1 {
      n140 = invoke class="VI" method="FP.Close"() -> ()  [unwired: 3 in, 3 out]
    }
  }
